vi "Test Suite Start Time.vi"(8 "error in (no error)":errorcluster, 11 "Test Suite Result Test In":refnum<class "Test Suite Result Test.lvclass">) -> (0 "error out":errorcluster, 3 "Test Suite Result Test Out":refnum<class "Test Suite Result Test.lvclass">)   [LabVIEW 2020, in "LUnit Tests.lvlib" / "Test Suite Result Test.lvclass"]
uses:
  Test Suite Result Test.lvclass
  C:/Program Files (x86)/National Instruments/LabVIEW 2020/vi.lib/Asteme/LUnit/Test Case.lvclass
  Test Dummys/Test Test Case/Test Test Case.lvclass
  C:/Users/anton/Documents/GitHub/LUnit/source/Framework/Test Case/LUnit Test Case.lvclass
  source/Framework/Result Classes/Test Suite Result/Test Suite Result.lvclass/Test Suite Result.ctl
  <vilib>/Asteme/LUnit/Test Case.lvclass/Test Case.ctl
  <vilib>/Asteme/LUnit/LUnit Assertion Result.lvclass/LUnit Assertion Result.ctl
  <vilib>/Asteme/LUnit/LUnit Test Case Result.lvclass/LUnit Test Case Result.ctl
  <vilib>/Asteme/LUnit/LUnit Method Result.lvclass/LUnit Method Result.ctl
  <vilib>/Asteme/LUnit/Palette/Fail.vi
  <vilib>/Asteme/LUnit/Palette/Pass.vi
  <vilib>/Asteme/LUnit/Set Assertion Type.vi
  <vilib>/Asteme/LUnit/Add test result.vi
  <vilib>/Asteme/LUnit/LUnit Write Passed.vi
  <vilib>/Asteme/LUnit/LUnit Write Message.vi
  <vilib>/Asteme/LUnit/LUnit Write Description.vi
  <vilib>/Asteme/LUnit/LUnit Write Assertion Type.vi
  <vilib>/Asteme/LUnit/LUnit Record Assertion Result.vi
  <vilib>/Asteme/LUnit/LUnit Aggregate Assertion Results.vi
  <vilib>/Asteme/LUnit/Assertion Result/LUnit Read Status.vi
  <vilib>/Asteme/LUnit/LUnit Read Message.vi
  <vilib>/Asteme/LUnit/LUnit Read Description.vi
  <vilib>/Asteme/LUnit/Method Result/LUnit Merge Status.vi
  <vilib>/Asteme/LUnit/LUnit Concatenate result strings.vi
  <vilib>/Asteme/LUnit/LUnit Assertion Result.lvclass
  <vilib>/Asteme/LUnit/Test Case.lvclass
  source/Framework/Result Classes/Test Suite Result/Test Suite Result.lvclass
  C:/Users/anton/Documents/GitHub/LUnit/tests/Test Dummys/Test Test Case/Test Test Case.lvclass
  C:/Users/anton/Documents/GitHub/LUnit/tests/Framework Test/Test Suite Result/Test Suite Result Test.lvclass
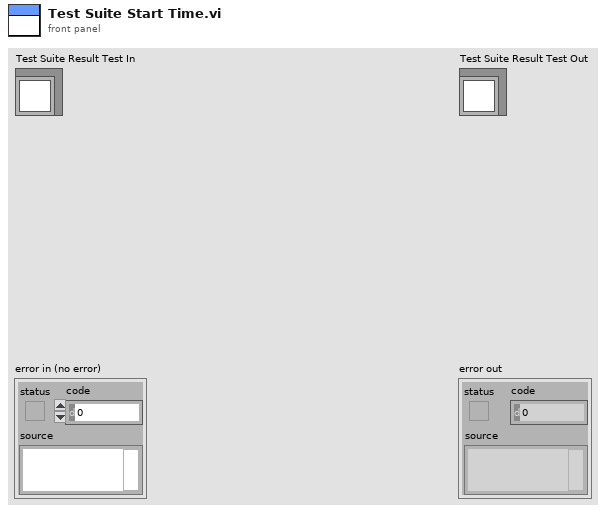
[diagram p1: front panel]
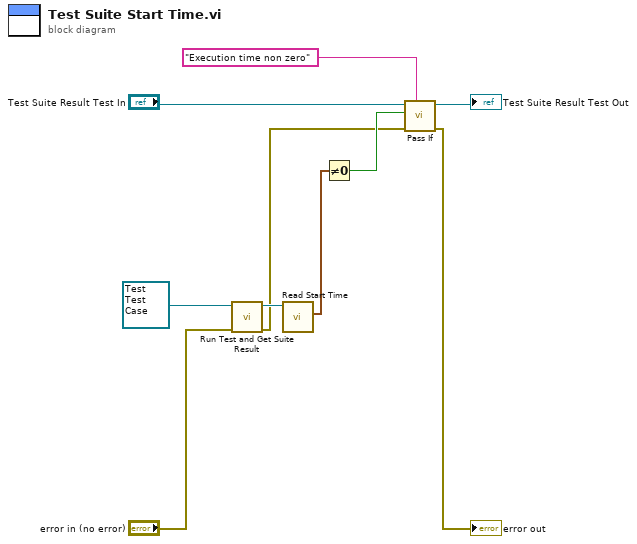
[diagram p0: block diagram]
diagram:
  n1 = call "Run Test and Get Suite Result.vi"("error in (no error)"="error in (no error)", "Test Test Case in"=refnum<class "Test Test Case.lvclass"> refnum ("Test Test Case.lvclass")) -> ("error out"=w1:errorcluster, "Test Suite Result out"=w4:refnum<class "Test Suite Result.lvclass">)  [unwired: 8 in]
  n2 = call "Read Start Time.vi"("Test Suite Result In"=w4) -> ("Start Time"=w6:timestamp)  [unwired: 9 in, 1 out]
  n3 = Not Equal To 0?(x=w6) -> (x != 0?=w5:bool)
  n4 = call <vilib>:"Pass If.vi"("Description"="Execution time non zero", "error in (no error)"=w1, "Pass?"=w5, "LUnit Test Case In"="Test Suite Result Test In") -> ("error out"=→"error out":errorcluster, "LUnit Test Case Out"=→"Test Suite Result Test Out":refnum<class "Test Suite Result Test.lvclass">)  [unwired: 6 in]
